vi "Scope Test.vi"(8 "error in (no error)":errorcluster) -> (0 "error out":errorcluster)   [LabVIEW 2020]
uses:
  G-Embedded-Python-Interpreter-Toolkit/G-Embedded-Python-Interpreter-Toolkit.lvlib
  <vilib>/addons/_JKI Toolkits/Caraya/classes/Test/Test.lvclass
  <vilib>/addons/_JKI Toolkits/Caraya/classes/Assert/Assert.lvclass
  <vilib>/addons/_JKI Toolkits/Caraya/classes/Assert/Assert Equal Value and Type_Variant.vi
panel:
  out "Value":i32
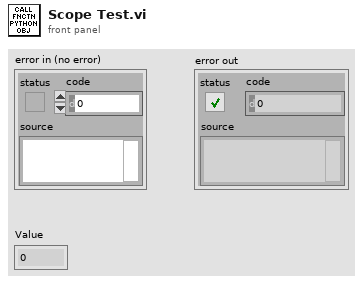
[diagram p1: front panel]
types:
  T1 = typedef "G-Embedded-Python-Interpreter-Toolkit.lvlib/Python Object Reference.ctl" = refnum<k1>
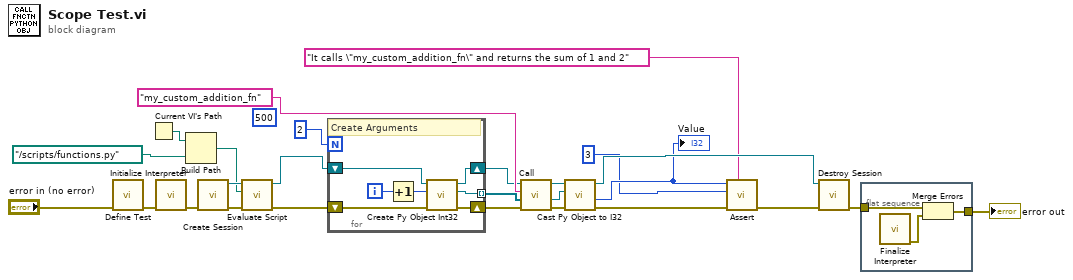
[diagram p0: block diagram]
diagram:
  (unwired) 500
  n1 = call <vilib>:"Define Test.vi"("error in (no error)"="error in (no error)") -> ("error out"=w26:errorcluster)  [unwired: 10 in]
  n2 = Current VI's Path() -> (path=w21:path)
  n3 = call "Initialize Interpreter.vi"("error in (no error)"=w26) -> ("error out"=w23:errorcluster)  [unwired: 9 in, 1 out]
  n4 = Build Path(base path=w21, name or relative path=path "../scripts/functions.py" ("Path")) -> (appended path=w19:path)
  n5 = call "Create Session.vi"("error in (no error)"=w23) -> ("error out"=w18:errorcluster, "Session Handle"=w22:refnum<data-value>)  [unwired: 9 in]
  n6 = call "Evaluate Script.vi"("error in (no error)"=w18, "Script File Path"=w19, "Session Handle in"=w22) -> ("error out"=w15:errorcluster, "Session Handle out"=w16:refnum<data-value>)  [unwired: 7 in]
  n7 = for {
    N: 2 -> [_]
    shift-right: [w29] -> w6
    shift-left: w16 -> [w33]
    shift-right: [w30] -> w7
    shift-left: w15 -> [w32]
    tunnel: [w28] -> w5 mode=indexing
    i -> [w31]
    # "Create Arguments"
    n8 = Increment(x=w31) -> (x+1=w27:i32)
    n9 = call "Create Py Object Int32.vi"("error in (no error)"=w32, "Value"=w27, "Session Handle in"=w33) -> ("error out"=w30:errorcluster, "Python Object Refnum"=w28:T1, "Session Handle out"=w29:refnum<data-value>)  [unwired: 6 in]
  }
  n10 = call "Call.vi"("error in (no error)"=w7, "Arguments"=w5, "Function/Method Name"="my_custom_addition_fn" ("Function Name"), "Session Handle in"=w6) -> ("error out"=w2:errorcluster, "Returned Python Object Refnum"=w3:T1, "Session Handle out"=w4:refnum<data-value>)  [unwired: 5 in]
  n11 = call "Cast Py Object to I32.vi"("error in (no error)"=w2, "Python Object Refnum in"=w3, "Session Handle in"=w4) -> ("error out"=w11:errorcluster, "Value"=w12:i32, "Session Handle out"=w13:refnum<data-value>)  [unwired: 5 in, 1 out]
  "Value" <- w12
  n12 = call-poly <vilib>:"Assert.vi"("Label"="It calls \"my_custom_addition_fn\" and returns the sum of 1 and 2", "error in (no error)"=w11, "Y"=3 ("Value"), "X"=w12) -> ("error out"=w10:errorcluster)  [unwired: 7 in]
  n13 = call "Destroy Session.vi"("error in (no error)"=w10, "Session Handle"=w13) -> ("error out"=w17:errorcluster)  [unwired: 9 in]
  n14 = flat-sequence {
    tunnel: w17 -> [w36]
    tunnel: [w34] -> w24
    frame #0 {
      n15 = call "Finalize Interpreter.vi"() -> ("error out"=w35:errorcluster)  [unwired: 11 in]
      n16 = Merge Errors(w36, w35) -> (w34:errorcluster)
    }
  }
  "error out" <- w24
